vi "GetTonePhase.vi"(2 "Selection":u8(ring) items=["Value", "Minimum", "Maximum"], 4 "error in (no error)":errorcluster, 5 "Tone Index":u16(ring) items=["Tone 1", "Tone 2", "Tone 3", "Tone 4", "Tone 5", "Tone 6", "Tone 7", "Tone 8", "Tone 9", "Tone 10"], 6 "ParamWave Name":string, 7 "VISA resource name":refnum<visa-resource-name>) -> (0 "error out":errorcluster, 1 "Phase  [°]":dbl, 3 "VISA resource name out":refnum<visa-resource-name>)   [LabVIEW 2020, in "Active Technologies AWG3000.lvlib"]
uses:
  Active Technologies AWG3000.lvlib
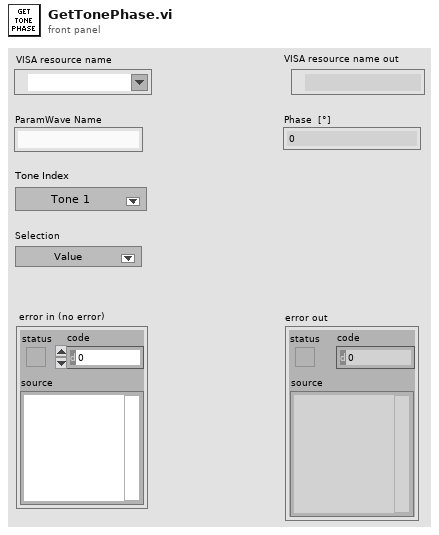
[diagram p1: front panel]
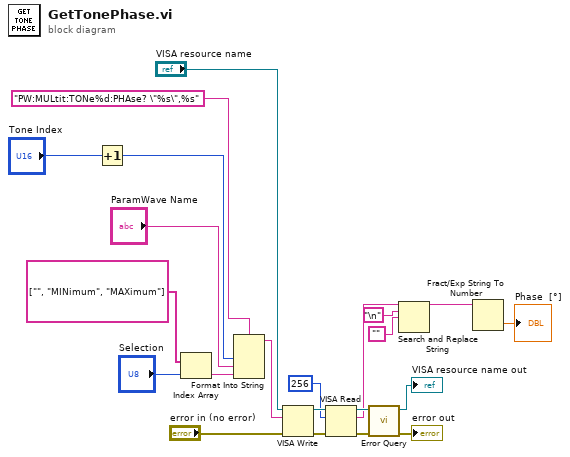
[diagram p0: block diagram]
diagram:
  n1 = Increment(x="Tone Index") -> (x+1=w2:u16)
  n2 = Index Array(array=string[] ["", "MINimum", "MAXimum"], index="Selection") -> (element=w5:string)
  n3 = Format Into String(format string="PW:MULtit:TONe%d:PHAse? \"%s\",%s" ("write buffer"), w2, "ParamWave Name", w5) -> (resulting string=w6:string)  [unwired: 2 in, 1 out]
  n4 = VISA Write(VISA resource name="VISA resource name", write buffer=w6, error in (no error)="error in (no error)") -> (VISA resource name out=w20:refnum<visa-resource-name>, error out=w19:errorcluster)  [unwired: 1 out]
  n5 = VISA Read(VISA resource name=w20, byte count=u32 256, error in (no error)=w19) -> (VISA resource name out=w17:refnum<visa-resource-name>, read buffer=w7:string, error out=w16:errorcluster)  [unwired: 1 out]
  n6 = call "Error Query.vi"("error in (no error)"=w16, "VISA resource name"=w17) -> ("error out"=→"error out":errorcluster, "VISA resource name out"=→"VISA resource name out":refnum<visa-resource-name>)  [unwired: 6 in, 2 out]
  n7 = Search and Replace String(input string=w7, search string="\n", replace string="") -> (result string=w10:string)  [unwired: 5 in, 3 out]
  n8 = Fract/Exp String To Number(string=w10) -> (number=→"Phase  [°]":dbl)  [unwired: 3 in, 1 out]
